vi "delete.vi"(7 "tree (dvr) in":refnum<data-value>, 8 "error in (no error)":errorcluster, 11 "Key":T1) -> (0 "error out":errorcluster, 2 "Found?":bool, 3 "Deleted?":bool)   [LabVIEW 2015, in "binary_tree.lvlib"]
uses:
  binary_tree.lvlib
  _Controls/node_key.ctl
  _Controls/tree.ctl
  _Controls/node_data.ctl
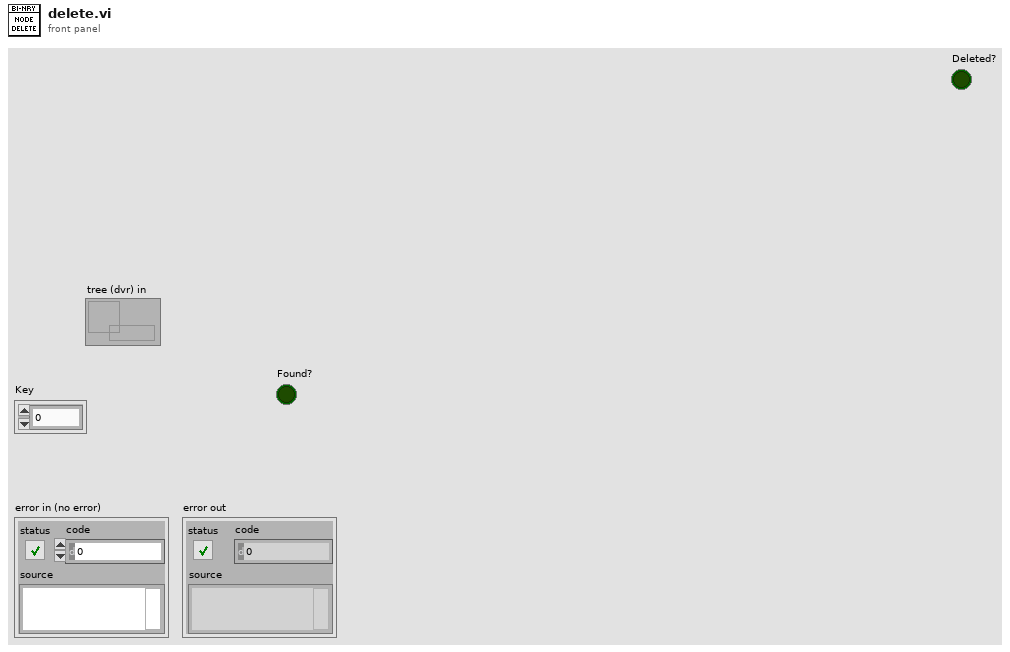
[diagram p1: front panel]
types:
  T1 = typedef "binary_tree.lvlib/node_key.ctl" = cluster{dbl}
  T2 = typedef "binary_tree.lvlib/tree.ctl" = cluster{"key":T1, "data":T3, "node_dvr (left)":variant, "node_dvr (right)":variant}
  T3 = typedef "binary_tree.lvlib/node_data.ctl" = cluster{dbl}
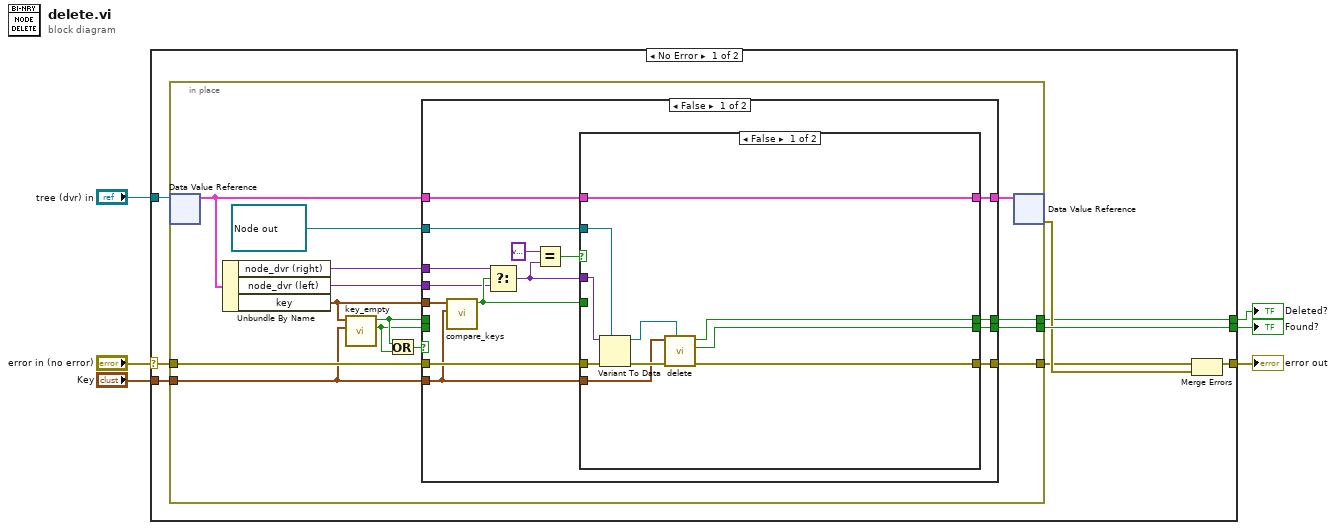
[diagram p0: block diagram]
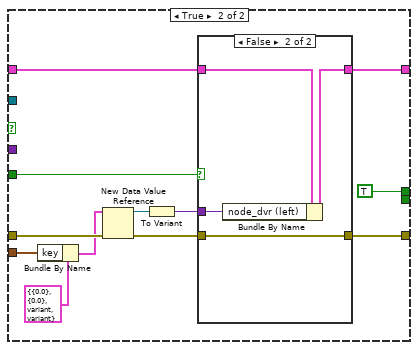
[diagram p2: hidden frame]
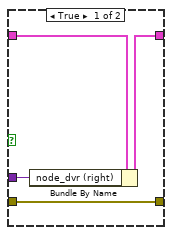
[diagram p3: hidden frame]
diagram:
  n1 = case shown="No Error" "error in (no error)" {
    selector: "error in (no error)" -> [w9 w78]
    tunnel: [w10 w78] -> w6
    tunnel: [w14 _] -> w2
    tunnel: "tree (dvr) in" -> [w13 _]
    tunnel: "Key" -> [w8 _]
    tunnel: [w7 _] -> w1
    frame No Error {
      n2 = in-place {
        in-place-border: w9 -> [w28]
        in-place-border: [w27] -> w11
        in-place-border: [w26] -> w14
        in-place-border: w8 -> [w17]
        in-place-border: [w22] -> w7
        n3 = in-place-dvr #1(w13) -> (w24:T2)  [unwired: 1 out]
        n4 = Unbundle By Name(w24) -> ("node_dvr (right)"=w21:variant, "node_dvr (left)"=w20:variant, "key"=w19:T1)
        n5 = call "key_empty.vi"("Key (search)"=w17, "Key (node)"=w19) -> ("Equal?"=w15:bool, "Empty?"=w16:bool)  [unwired: 8 in]
        n6 = Or(x=w16, y=w15) -> (x .or. y?=w18:bool)
        n7 = case shown="False" w18 {
          tunnel: w19 -> [w43 _]
          tunnel: w28 -> [w42 w75]
          tunnel: [w40 w75] -> w27
          tunnel: [w39 w76] -> w26
          tunnel: refnum<data-value> refnum ("tree (dvr)") -> [w38 _]
          tunnel: w24 -> [w37 w74]
          tunnel: [w36 w74] -> w23
          tunnel: w17 -> [w35 _]
          tunnel: [w33 w77] -> w22
          tunnel: w21 -> [w32 _]
          tunnel: w20 -> [w31 _]
          tunnel: w16 -> [_ w77]
          tunnel: w15 -> [_ w76]
          frame False {
            n8 = call "compare_keys.vi"("Key (search)"=w35, "Key (node)"=w43) -> ("Left(F)/Right(T)"=w34:bool)  [unwired: 8 in, 1 out]
            n9 = Select(t=w32, s=w34, f=w31) -> (s? t:f=w41:variant)
            n10 = Equal?(x=variant ("Left"), y=w41) -> (x = y?=w30:bool)
            n11 = case shown="False" w30 {
              tunnel: w42 -> [w53 w65]
              tunnel: w41 -> [w52 _]
              tunnel: [w50 w55] -> w40
              tunnel: [w44 _] -> w39
              tunnel: w38 -> [w48 _]
              tunnel: w35 -> [w47 w61]
              tunnel: w37 -> [w46 w62]
              tunnel: [w46 w57] -> w36
              tunnel: w34 -> [_ w59]
              tunnel: [w45 TRUE] -> w33
              frame False {
                n12 = Variant To Data(error in=w53, type=w48, Variant=w52) -> (data=w49:refnum<data-value>, error out=w51:errorcluster)
                n13 = call "delete.vi"("tree (dvr) in"=w49, "error in (no error)"=w51, "Key"=w47) -> ("error out"=w50:errorcluster, "Found?"=w44:bool, "Deleted?"=w45:bool)  [unwired: 6 in]
              }
              frame True {
                n14 = Bundle By Name(cluster=T2 {"key"={0.0}, "data"={0.0}, "node_dvr (left)"=variant, "node_dvr (right)"=variant} ("data value"), "key"=w61) -> (w64:T2)
                n15 = New Data Value Reference(data value=w64, error in=w65) -> (data value reference=w60:refnum<data-value>, error out=w56:errorcluster)
                n16 = To Variant(anything=w60) -> (Variant=w58:variant)
                n17 = case shown="False" w59 {
                  tunnel: w62 -> [w69 w73]
                  tunnel: w58 -> [w68 w72]
                  tunnel: [w67 w71] -> w57
                  tunnel: w56 -> [w66 w70]
                  tunnel: [w66 w70] -> w55
                  frame True {
                    n18 = Bundle By Name(cluster=w69, "node_dvr (right)"=w68) -> (w67:T2)
                  }
                  frame False {
                    n19 = Bundle By Name(cluster=w73, "node_dvr (left)"=w72) -> (w71:T2)
                  }
                }
              }
            }
          }
          frame True {
          }
        }
        n20 = in-place-dvr #1(w23) -> (w12:errorcluster)  [unwired: 1 out]
      }
      n21 = Merge Errors(w11, w12) -> (w10:errorcluster)
    }
    frame Error {
    }
  }
  "error out" <- w6
  "Found?" <- w2
  "Deleted?" <- w1
